vi "Exit With Error Cluster Code.vi"(8 "error in (no error)":errorcluster, 10 "No Error Code (0)":i32, 11 "CLI in":refnum<class "CLI.lvclass">) -> (0 "error out":errorcluster)   [LabVIEW 2015, in "CLI.lvclass"]
doc: "Exits the interface using the error cluster to determine the exit code.\n\nIf <b>error in</b> has an error this code is returned and the error message from LabVIEW.\n\nIf there is no error, exit with code 0."
uses:
  CLI.lvclass
  <vilib>/Utility/error.llb/DialogType.ctl
  Output.ctl
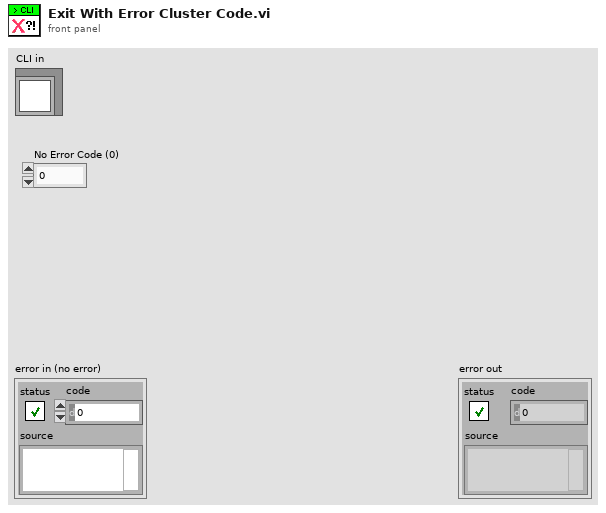
[diagram p1: front panel]
types:
  T1 = typedef "CLI.lvclass/Output.ctl" = enum16{"StdOut", "StdErr"}
  T2 = typedef "DialogType.ctl" = u16
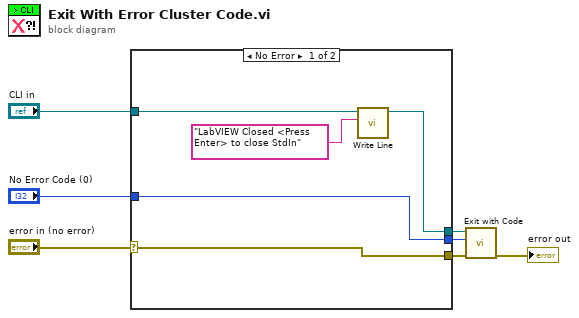
[diagram p0: block diagram]
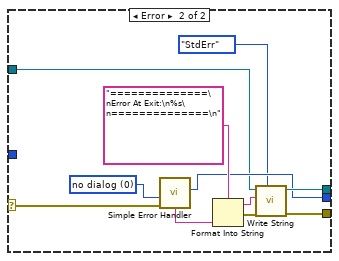
[diagram p2: hidden frame]
diagram:
  n1 = case shown="No Error" "error in (no error)" {
    selector: "error in (no error)" -> [w12 w14]
    tunnel: [w12 w23] -> w7
    tunnel: [w9 w22] -> w6
    tunnel: [w11 w17] -> w4
    tunnel: "CLI in" -> [w10 w15]
    tunnel: "No Error Code (0)" -> [w11 _]
    frame No Error {
      n2 = call "Write Line.vi"("Text to Write"="LabVIEW Closed <Press Enter> to close StdIn", "CLI in"=w10) -> ("CLI out"=w9:refnum<class "CLI.lvclass">)  [unwired: 8 in, 1 out]
    }
    frame Error {
      w21 = T2 0 items=["no dialog", "OK message", "continue or stop message", "OK message + warnings", "continue/stop + warnings"] ("type of dialog (OK msg:1)")
      n3 = call <vilib>:"Simple Error Handler.vi"("type of dialog (OK msg:1)"=w21, "error in (no error)"=w14) -> ("code out"=w17:i32, "message"=w18:string)  [unwired: 3 in, 3 out]
      n4 = Format Into String(format string="==============\nError At Exit:\n%s\n==============\n", w18) -> (resulting string=w16:string, error out=w20:errorcluster)  [unwired: 2 in]
      n5 = call "Write String.vi"("Output (StdOut)"=Output."StdErr", "error in (no error)"=w20, "Text to Write"=w16, "CLI in"=w15) -> ("error out"=w23:errorcluster, "CLI out"=w22:refnum<class "CLI.lvclass">)  [unwired: 6 in]
    }
  }
  n6 = call "Exit with Code.vi"("error in (no error)"=w7, "Exit Code (0)"=w4, "CLI in"=w6) -> ("error out"=→"error out":errorcluster)  [unwired: 8 in]
